vi "_ROSMasterConsole.vi"() -> ()   [LabVIEW 2012]
uses:
  Program Files (x86)/National Instruments/LabVIEW 2013/user.lib/ROSforLV/ROS/Code/_ROSDefinition.vi
  <vilib>/Utility/miscctls.llb/LVRectTypeDef.ctl
  <vilib>/Utility/cursorutil.llb/Set Cursor (Icon Pict).vi
panel:
  in  "Ping":bool
  in  "Delete servers on close":bool=TRUE
  out "Servers Closed":bool[](array[boolean])
  in  "Stop":bool
  out "Error Log":string
  out "ROS Master":string="192.168.1.110:11311"
  out "selection":i32=-1
  out "2D Picture":picture
  out "Boundaries":cluster{i32, i32}[](array[cluster])=[{10, 22}, {30, 42}, {50, 62}]
  in  "expand?":bool
  out "Status":string
  out "Connections":bool
  out "Master?":bool
  out "Running?":bool
  out "current task":string
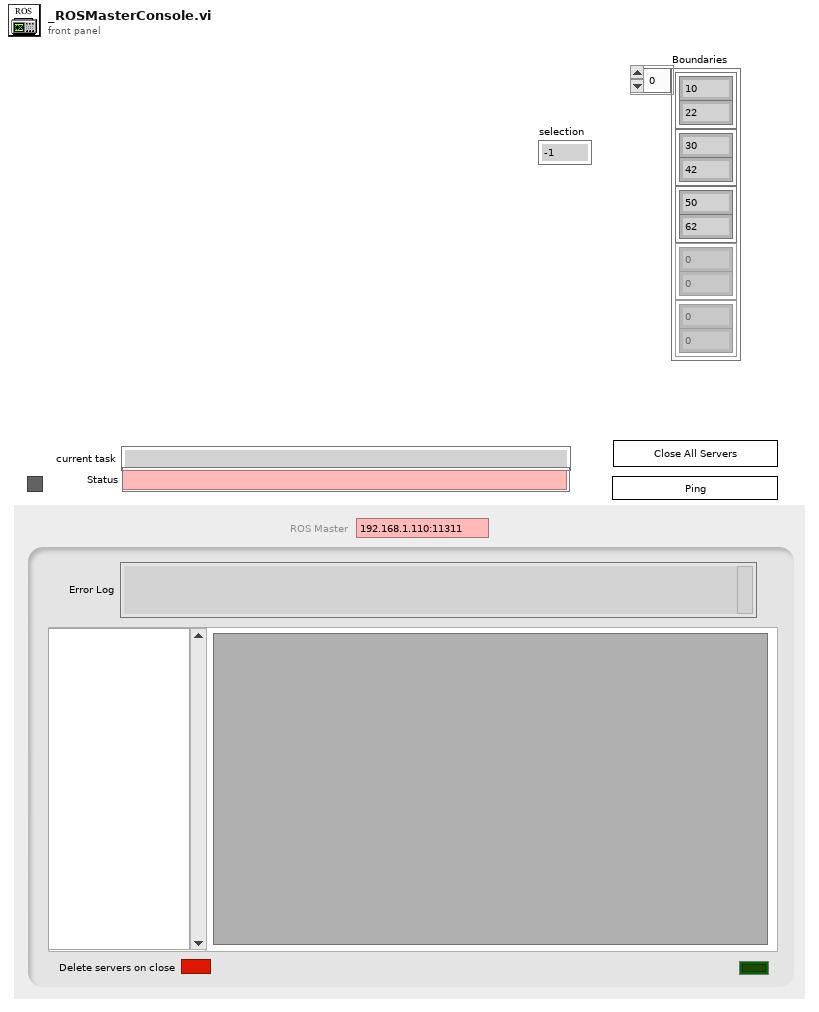
[diagram p1: front panel]
types:
  T1 = enum16{"Add Server", "Clear Server", "Clear All", "Get Info"}
  T2 = enum16{"Get Nodes", "Start Nodes", "Reset Nodes"}
  T3 = typedef "LVRectTypeDef.ctl" = cluster{"Left":i16, "Top":i16, "Right":i16, "Bottom":i16}
  T4 = typedef "_ROSControl.ctl" = cluster{"topic port":u16, "Node":string, "topic":string, "type":string, "node port":u32, "error ":errorcluster, "Direction":T5, "APIs":string[], "Update (ms)":u16, "write queue":u16}
  T5 = typedef "_ROSDirection.ctl" = enum16{"Node", "Publisher", "Subscriber", "Service Client"}
  T6 = typedef "ServoInfo.ctl" = cluster{"vi name":string, "VI Refnum":refnum<vi>, "queue":refnum<queue>, "ROS":T4, "notifier":refnum<notifier>}
  T7 = enum32{"Invalid", "Standard", "Closed", "Hidden", "Minimized", "Maximized"}
  T8 = typedef "LVMouseTypeDef.ctl" = cluster{"Mouse Position":cluster{"X":i32, "Y":i32}, "Mouse Modifiers":cluster{"Button Down":bool, "Shift Mod":bool, "Menu Mod":bool, "Option Mod":bool}}
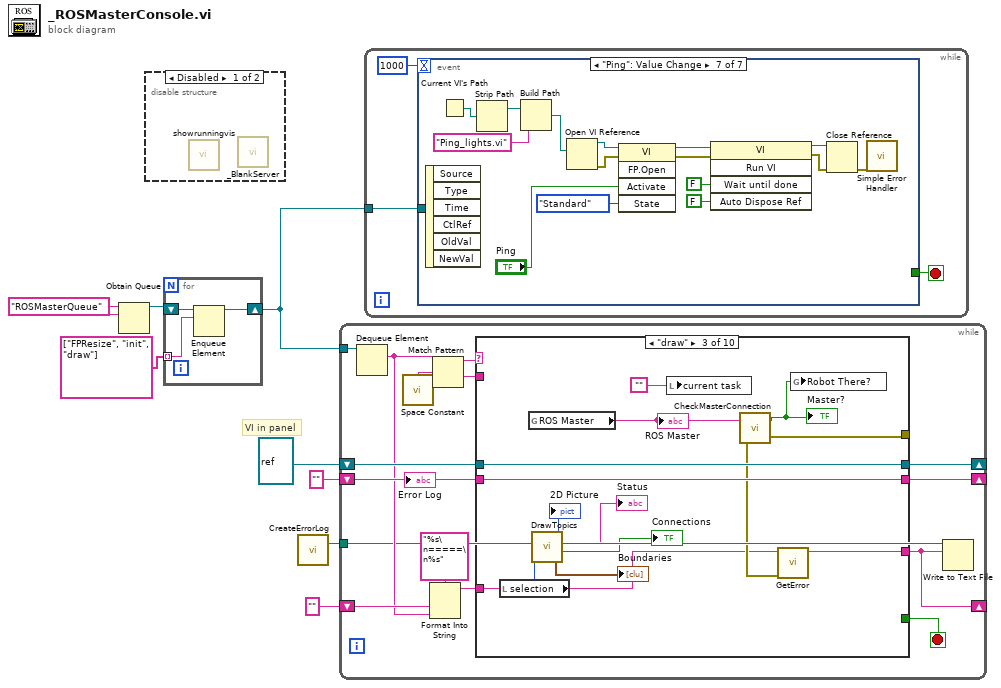
[diagram p0: block diagram]
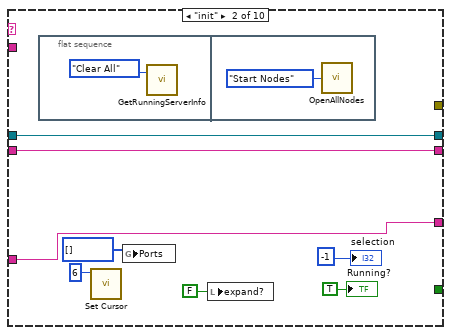
[diagram p4: hidden frame]
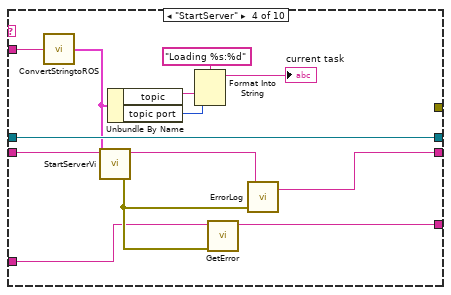
[diagram p5: hidden frame]
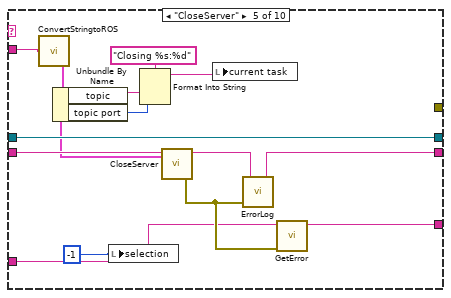
[diagram p6: hidden frame]
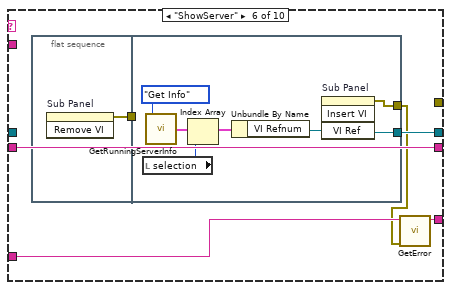
[diagram p7: hidden frame]
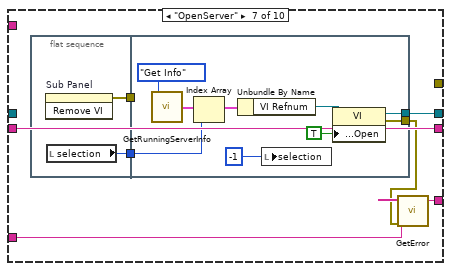
[diagram p8: hidden frame]
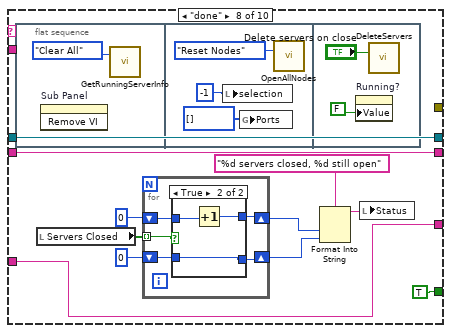
[diagram p9: hidden frame]
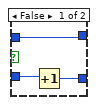
[diagram p10: hidden frame]
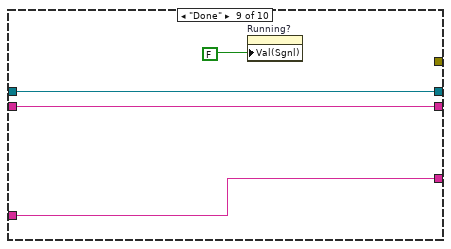
[diagram p11: hidden frame]
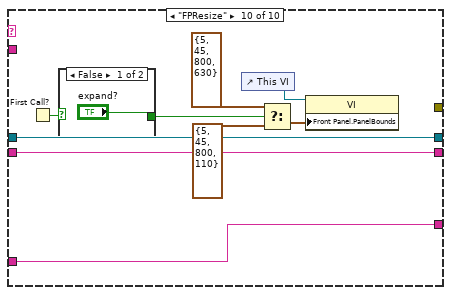
[diagram p12: hidden frame]
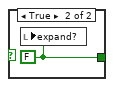
[diagram p13: hidden frame]
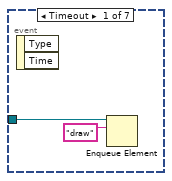
[diagram p14: hidden frame]
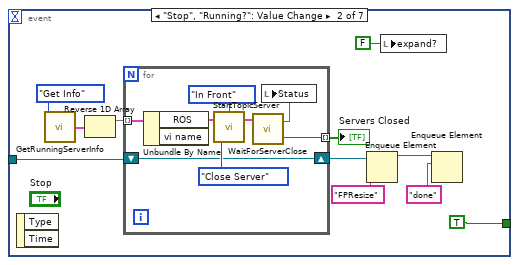
[diagram p15: hidden frame]
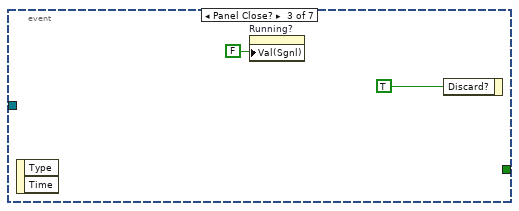
[diagram p16: hidden frame]
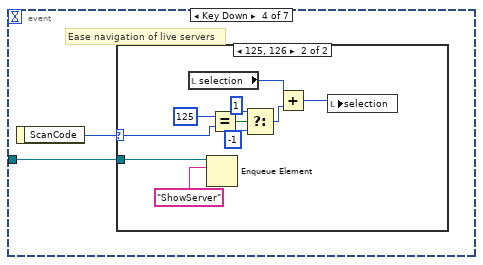
[diagram p17: hidden frame]
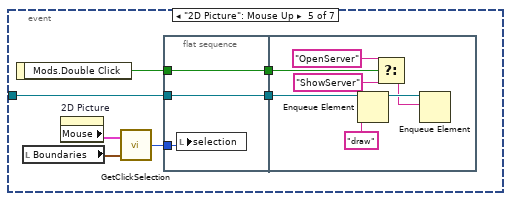
[diagram p19: hidden frame]
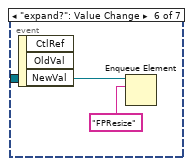
[diagram p20: hidden frame]
diagram:
  w8 = "ROSMasterQueue" ("name (unnamed)")
  # "VI in panel"
  n1 = Obtain Queue(name (unnamed)=w8, element data type=w8) -> (queue out=w5:refnum<queue>)  [unwired: 3 in, 2 out]
  n2 = disable-structure shown="Disabled" {
    frame Disabled {
      n3 = call "showrunningvis.vi"() -> ()  [unwired: 1 in]
      n4 = call "_BlankServer.vi"() -> ()  [unwired: 4 in]
    }
    frame Enabled {
    }
  }
  n5 = for {
    shift-right: [w11] -> w7
    shift-left: w5 -> [w10]
    tunnel: string[] ["FPResize", "init", "draw"] -> [w9] mode=indexing
    n6 = Enqueue Element(queue=w10, element=w9) -> (queue out=w11:refnum<queue>)  [unwired: 2 in, 2 out]
  }
  n7 = call "CreateErrorLog.vi"() -> ("path"=w1:path)  [unwired: 11 in]
  n8 = while {
    tunnel: w7 -> [w26]
    shift-right: [w20] -> _
    shift-left: refnum<vi> refnum ("VI Ref") -> [w21]
    shift-right: [w19] -> _
    shift-left: "" ("String out") -> [w18]
    shift-right: [w13] -> _
    shift-left: "" -> [w17]
    tunnel: w1 -> [w12]
    stop <- w25 stop-if-true
    n9 = Dequeue Element(queue=w26) -> (element=w15:string)  [unwired: 2 in, 3 out]
    n10 = call <vilib>:"Space Constant.vi"() -> ("String"=w23:string)
    n11 = Format Into String(format string="%s\n=====\n%s", w17, w15) -> (resulting string=w14:string)  [unwired: 2 in, 1 out]
    n12 = Match Pattern(string=w15, regular expression=w23) -> (before substring=w24:string, after substring=w22:string)  [unwired: 1 in, 2 out]
    n13 = case shown="\"draw\"" w24 {
      tunnel: [_ _ _ _ _ _ _ TRUE _ _] -> w25
      tunnel: w22 -> [_ _ _ w61 w70 _ _ _ _ _]
      tunnel: w21 -> [w29 w37 w52 w64 w77 _ _ w118 w140 w149]
      tunnel: [w29 w37 w52 w64 w77 w82 w95 w118 w140 w149] -> w20
      tunnel: [_ _ w44 _ _ _ _ _ _ _] -> _
      tunnel: [w28 w31 w48 w56 w74 w81 w94 w117 w138 w142] -> w19
      tunnel: w18 -> [w28 w31 w48 w57 w75 w81 w94 w117 w138 w142]
      tunnel: w14 -> [w27 w30 w43 w54 w65 w79 w92 w109 w137 w141]
      tunnel: [w27 w30 w42 w53 w67 w80 w93 w109 w137 w141] -> w13
      frame Default {
      }
      frame "init" {
        n14 = flat-sequence {
          frame #0 {
            n15 = call "GetRunningServerInfo.vi"("Task"=T1."Clear All") -> ()  [unwired: 1 in, 3 out]
          }
          frame #1 {
            n16 = call "OpenAllNodes.vi"("Task"=T2."Start Nodes") -> ()  [unwired: 1 in, 1 out]
          }
        }
        n17 = call-poly <vilib>:"Set Cursor.vi"("icon"=u16 6) -> ()  [unwired: 9 in, 2 out]
        n18 = global write "_ROSDefinition.vi" "Ports"(u16[] [] ("Ports")) -> ()
        n19 = local write "expand?"(FALSE ("expand?")) -> ()
        "Running?" <- TRUE ("Running?")
        "selection" <- -1 ("selection")
      }
      frame "draw" {
        n20 = local read "selection"() -> (w51:i32)
        n21 = global read "_ROSDefinition.vi" "ROS Master"() -> (w46:string)
        "ROS Master" <- w46
        n22 = call "DrawTopics.vi"("Selection"=w51) -> ("new picture"=→"2D Picture":picture, "Status"=→"Status":string, "all good?"=→"Connections":bool, "Boundaries"=→"Boundaries":cluster{i32, i32}[])  [unwired: 2 in]
        n23 = local write "current task"("") -> ()
        n24 = call "CheckMasterConnection.vi"("Master IP"=w46) -> ("error out"=w44:errorcluster, "Master There?"=w45:bool)  [unwired: 1 in]
        "Master?" <- w45
        n25 = call "GetError.vi"("error in (no error)"=w44, "String in"=w43) -> ("String out"=w42:string)  [unwired: 9 in]
        n26 = global write "_ROSDefinition.vi" "Robot There?"(w45) -> ()
      }
      frame "StartServer" {
        n27 = call "ConvertStringtoROS.vi"("string in"=w61) -> ("ROS"=w58:T4)
        n28 = call "StartServerVi.vi"("ROS in"=w58) -> ("error out"=w55:errorcluster)  [unwired: 2 out]
        n29 = Unbundle By Name(w58) -> ("topic"=w60:string, "topic port"=w59:u16)
        n30 = Format Into String(format string="Loading %s:%d", w60, w59) -> (resulting string=→"current task":string)  [unwired: 2 in, 1 out]
        n31 = call "GetError.vi"("error in (no error)"=w55, "String in"=w54) -> ("String out"=w53:string)  [unwired: 9 in]
        n32 = call "ErrorLog.vi"("error in"=w55, "String in"=w57) -> ("String out"=w56:string)  [unwired: 1 in, 1 out]
      }
      frame "CloseServer" {
        n33 = call "ConvertStringtoROS.vi"("string in"=w70) -> ("ROS"=w68:T4)
        n34 = Unbundle By Name(w68) -> ("topic"=w72:string, "topic port"=w71:u16)
        n35 = local write "selection"(-1 ("Value (Signaling)")) -> ()
        n36 = Format Into String(format string="Closing %s:%d", w72, w71) -> (resulting string=w69:string)  [unwired: 2 in, 1 out]
        n37 = call "CloseServer.vi"("ROS"=w68) -> ("error out"=w66:errorcluster)  [unwired: 2 in]
        n38 = local write "current task"(w69) -> ()
        n39 = call "ErrorLog.vi"("error in"=w66, "String in"=w75) -> ("String out"=w74:string)  [unwired: 1 in, 1 out]
        n40 = call "GetError.vi"("error in (no error)"=w66, "String in"=w65) -> ("String out"=w67:string)  [unwired: 9 in]
      }
      frame "ShowServer" {
        n41 = flat-sequence {
          tunnel: [w84] -> w83
          tunnel: w83 -> [_]
          tunnel: [w90] -> w78
          tunnel: [w85] -> w82
          frame #0 {
            n42 = invoke on="Sub Panel" class="SubPanel" method="Remove VI"() -> (error out=w84:errorcluster)  [unwired: 3 in, 2 out]
          }
          frame #1 {
            n43 = local read "selection"() -> (w89:i32)
            n44 = call "GetRunningServerInfo.vi"("Task"=T1."Get Info") -> ("servers"=w87:T6[])  [unwired: 1 in, 2 out]
            n45 = Index Array(array=w87, index=w89) -> (element=w86:T6)
            n46 = Unbundle By Name(w86) -> ("VI Refnum"=w85:refnum<vi>)
            n47 = invoke on="Sub Panel" class="SubPanel" method="Insert VI"("VI Ref"=w85) -> (error out=w90:errorcluster)  [unwired: 3 in, 3 out]
          }
        }
        n48 = call "GetError.vi"("error in (no error)"=w78, "String in"=w79) -> ("String out"=w80:string)  [unwired: 9 in]
      }
      frame "OpenServer" {
        n49 = flat-sequence {
          tunnel: [w99] -> w97
          tunnel: [w98] -> w96
          tunnel: w97 -> [_]
          tunnel: w96 -> [w101]
          tunnel: [w106] -> w95
          tunnel: [w105] -> w91
          frame #0 {
            n50 = invoke on="Sub Panel" class="SubPanel" method="Remove VI"() -> (error out=w99:errorcluster)  [unwired: 3 in, 2 out]
            n51 = local read "selection"() -> (w98:i32)
          }
          frame #1 {
            n52 = call "GetRunningServerInfo.vi"("Task"=T1."Get Info") -> ("servers"=w103:T6[])  [unwired: 1 in, 2 out]
            n53 = Index Array(array=w103, index=w101) -> (element=w102:T6)
            n54 = Unbundle By Name(w102) -> ("VI Refnum"=w100:refnum<vi>)
            n55 = local write "selection"(-1 ("Live Servers")) -> ()
            n56 = property class="VI"(reference=w100, "Front Panel.Open"=TRUE ("Front Panel Window:Open")) -> (reference out=w106:refnum<vi>, error out=w105:errorcluster)  [unwired: 1 in]
          }
        }
        n57 = call "GetError.vi"("error in (no error)"=w91, "String in"=w92) -> ("String out"=w93:string)  [unwired: 9 in]
      }
      frame "done" {
        n58 = flat-sequence {
          frame #0 {
            n59 = invoke on="Sub Panel" class="SubPanel" method="Remove VI"() -> ()  [unwired: 3 in, 3 out]
            n60 = call "GetRunningServerInfo.vi"("Task"=T1."Clear All") -> ()  [unwired: 1 in, 3 out]
          }
          frame #1 {
            n61 = local write "selection"(-1 ("Live Servers")) -> ()
            n62 = global write "_ROSDefinition.vi" "Ports"(u16[] [] ("Ports")) -> ()
            n63 = call "OpenAllNodes.vi"("Task"=T2."Reset Nodes") -> ()  [unwired: 1 in, 1 out]
          }
          frame #2 {
            n64 = property on="Running?" class="Bool (strict)"("Value"=FALSE) -> ()  [unwired: 2 in, 2 out]
            n65 = call "DeleteServers.vi"("Delete servers on close"="Delete servers on close") -> ()  [unwired: 3 in]
          }
        }
        n66 = local read "Servers Closed"() -> (w116:bool[])
        n67 = for {
          shift-right: [w128] -> w112
          shift-left: 0 -> [w129]
          shift-right: [w126] -> w111
          shift-left: 0 -> [w127]
          tunnel: w116 -> [w130] mode=indexing
          n68 = case shown="True" w130 {
            tunnel: w129 -> [w131 w136]
            tunnel: [w131 w135] -> w128
            tunnel: w127 -> [w133 w134]
            tunnel: [w132 w134] -> w126
            frame False {
              n69 = Increment(x=w133) -> (x+1=w132:i32)
            }
            frame True {
              n70 = Increment(x=w136) -> (x+1=w135:i32)
            }
          }
        }
        n71 = Format Into String(format string="%d servers closed, %d still open", w112, w111) -> (resulting string=w110:string)  [unwired: 2 in, 1 out]
        n72 = local write "Status"(w110) -> ()
      }
      frame "Done" {
        n73 = property on="Running?" class="Bool (strict)"("Val(Sgnl)"=FALSE) -> ()  [unwired: 2 in, 2 out]
      }
      frame "FPResize" {
        n74 = First Call?() -> (First Call?: T/F=w144:bool)
        n75 = case shown="False" w144 {
          tunnel: ["expand?" w151] -> w143
          frame False {
          }
          frame True {
            w151 = FALSE ("expand?")
            n76 = local write "expand?"(w151) -> ()
          }
        }
        n77 = control-ref of="This VI"() -> (w148:refnum<vi>)
        n78 = Select(t=T3 {"Left"=5, "Top"=45, "Right"=800, "Bottom"=630} ("Front Panel Window:Panel Bounds"), s=w143, f=T3 {"Left"=5, "Top"=45, "Right"=800, "Bottom"=110} ("Front Panel Window:Panel Bounds")) -> (s? t:f=w146:T3)
        n79 = property class="VI"(reference=w148, "Front Panel.PanelBounds"=w146) -> ()  [unwired: 1 in, 2 out]
      }
    }
    n80 = Write to Text File(file (use dialog)=w12, text=w13) -> ()  [unwired: 2 in, 3 out]
    "Error Log" <- w18
  }
  n81 = while {
    tunnel: w7 -> [w154]
    stop <- w153 stop-if-true
    n82 = event shown="[6] \"Ping\": Value Change" {
      selector: _ -> [_ _ _ _ _ _ _]
      dyn-events: _ -> [_ _ _ _ _ _ _]
      timeout: 1000 -> [_ _ _ _ _ _ _]
      tunnel: w154 -> [w156 w166 _ w179 w196 w207 _]
      tunnel: [_ TRUE ("Stop") _ _ _ _ _] -> w153
      event Timeout {
        n83 = event-data() -> ()  [unwired: 1 in, 2 out]
        n84 = Enqueue Element(queue=w156, element="draw") -> ()  [unwired: 2 in, 3 out]
      }
      event "Stop", "Running?": Value Change {
        n85 = event-data() -> ()  [unwired: 1 in, 2 out]
        n86 = call "GetRunningServerInfo.vi"("Task"=T1."Get Info") -> ("servers"=w158:T6[])  [unwired: 1 in, 2 out]
        n87 = Reverse 1D Array(array=w158) -> (reversed array=w159:T6[])
        n88 = for {
          shift-right: [w171] -> w163
          shift-left: w166 -> [w171]
          tunnel: w159 -> [w175] mode=indexing
          tunnel: [w168] -> w157 mode=indexing
          n89 = Unbundle By Name(w175) -> ("ROS"=w172:T4)  [unwired: 1 out]
          n90 = call "StartTopicServer.vi"("Server Direction"=enum16{"Start Server", "Close Server"}."Close Server", "ROS in"=w172, "Priority"=enum16{"In Front", "In Back"}."In Front") -> ("ROS out"=w170:T4)  [unwired: 1 in]
          n91 = call "WaitForServerClose.vi"("ROS in"=w170) -> ("Closed"=w168:bool, "resulting string"=w169:string)  [unwired: 1 in]
          n92 = local write "Status"(w169) -> ()
        }
        "Servers Closed" <- w157
        n93 = Enqueue Element(queue=w163, element="FPResize") -> (queue out=w162:refnum<queue>)  [unwired: 2 in, 2 out]
        n94 = local write "expand?"(FALSE ("expand?")) -> ()
        n95 = Enqueue Element(queue=w162, element="done") -> ()  [unwired: 2 in, 3 out]
      }
      event Panel Close? {
        n96 = event-data() -> ()  [unwired: 1 in, 2 out]
        n97 = property on="Running?" class="Bool (strict)"("Val(Sgnl)"=FALSE ("Value (Signaling)")) -> ()  [unwired: 2 in, 2 out]
        n98 = event-data("Discard?"=TRUE ("Stop")) -> ()  [unwired: 1 in, 1 out]
      }
      event Key Down {
        # "Ease navigation of live servers"
        n99 = event-data() -> ("ScanCode"=w178:i16)  [unwired: 1 in]
        n100 = case shown="125, 126" w178 {
          selector: w178 -> [_ w187]
          tunnel: w179 -> [_ w189]
          frame Default {
          }
          frame 125, 126 {
            n101 = local read "selection"() -> (w180:i32)
            n102 = Enqueue Element(queue=w189, element="ShowServer") -> ()  [unwired: 2 in, 3 out]
            n103 = Equal?(x=i16 125, y=w187) -> (x = y?=w185:bool)
            n104 = Select(t=i16 1 ("x"), s=w185, f=i16 -1 ("x")) -> (s? t:f=w184:i16)
            n105 = Add(x=w180, y=w184) -> (x+y=w181:i32)
            n106 = local write "selection"(w181) -> ()
          }
        }
      }
      event "2D Picture": Mouse Up {
        n107 = event-data() -> ("Mods.Double Click"=w193:bool)  [unwired: 1 in]
        n108 = local read "Boundaries"() -> (w194:cluster{i32, i32}[])
        n109 = property on="2D Picture" class="Pict"() -> ("Mouse"=w195:T8)  [unwired: 2 in, 2 out]
        n110 = call "GetClickSelection.vi"("Boundaries"=w194, "Mouse"=w195) -> ("selection"=w190:i32)
        n111 = flat-sequence {
          tunnel: w193 -> [w198]
          tunnel: w196 -> [w199]
          tunnel: [w199] -> w192
          tunnel: [w198] -> w191
          tunnel: w190 -> [w197]
          tunnel: w192 -> [w205]
          tunnel: w191 -> [w204]
          frame #0 {
            n112 = local write "selection"(w197) -> ()
          }
          frame #1 {
            n113 = Enqueue Element(queue=w205, element="draw" ("name (unnamed)")) -> (queue out=w201:refnum<queue>)  [unwired: 2 in, 2 out]
            n114 = Select(t="OpenServer" ("element"), s=w204, f="ShowServer" ("element")) -> (s? t:f=w200:string)
            n115 = Enqueue Element(queue=w201, element=w200) -> ()  [unwired: 2 in, 3 out]
          }
        }
      }
      event "expand?": Value Change {
        n116 = event-data() -> ()  [unwired: 1 in, 3 out]
        n117 = Enqueue Element(queue=w207, element="FPResize") -> ()  [unwired: 2 in, 3 out]
      }
      event "Ping": Value Change {
        n118 = event-data() -> ()  [unwired: 1 in, 6 out]
        n119 = Current VI's Path() -> (path=w222:path)
        n120 = Strip Path(path=w222) -> (stripped path=w223:path)  [unwired: 1 out]
        n121 = Build Path(base path=w223, name or relative path="Ping_lights.vi") -> (appended path=w219:path)
        n122 = Open VI Reference(vi path=w219) -> (vi reference=w220:refnum<vi>, error out=w216:errorcluster)  [unwired: 5 in]
        n123 = invoke class="VI" method="FP.Open"(reference=w220, error in=w216, "Activate"="Ping", "State"=T7."Standard") -> (reference out=w218:refnum<vi>, error out=w217:errorcluster)  [unwired: 1 in, 3 out]
        n124 = invoke class="VI" method="Run VI"(reference=w218, error in=w217, "Wait until done"=FALSE ("Wait Until Done"), "Auto Dispose Ref"=FALSE ("Auto Dispose Reference")) -> (reference out=w212:refnum<vi>, error out=w213:errorcluster)  [unwired: 1 in, 3 out]
        n125 = Close Reference(reference=w212, error in (no error)=w213) -> (error out=w211:errorcluster)
        n126 = call <vilib>:"Simple Error Handler.vi"("error in (no error)"=w211) -> ()  [unwired: 4 in, 5 out]
      }
    }
  }
